vi "Stringfunction.vi"() -> ()   [LabVIEW 2020]
panel:
  out "decimated array 5":dbl[](array[numeric])
  out "decimated array 4":dbl[](array[numeric])
  out "decimated array 3":dbl[](array[numeric])
  out "decimated array 2":dbl[](array[numeric])
  out "decimated array":dbl[](array[numeric])
  out "interleaved array":dbl[](array[numeric])
  out "appended array":dbl[][](array[numeric])
  out "array w/ subset deleted":dbl[][](array[numeric])
  out "output array 4":dbl[][](array[numeric])
  out "output array":dbl[][](array[numeric])
  out "min index(es)":i32[](array[numeric])
  out "max index(es)":i32[](array[numeric])
  out "size(s)":i32[](array[numeric])
  out "output array 3":dbl[][](array[numeric])
  out "min value":dbl
  out "max value":dbl
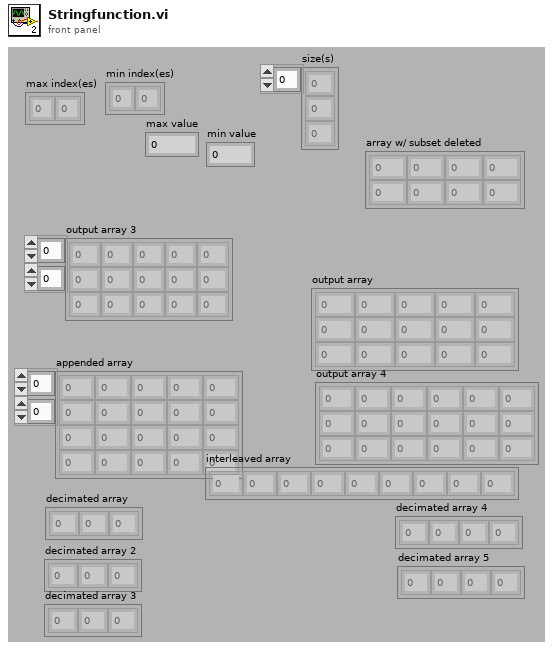
[diagram p1: front panel]
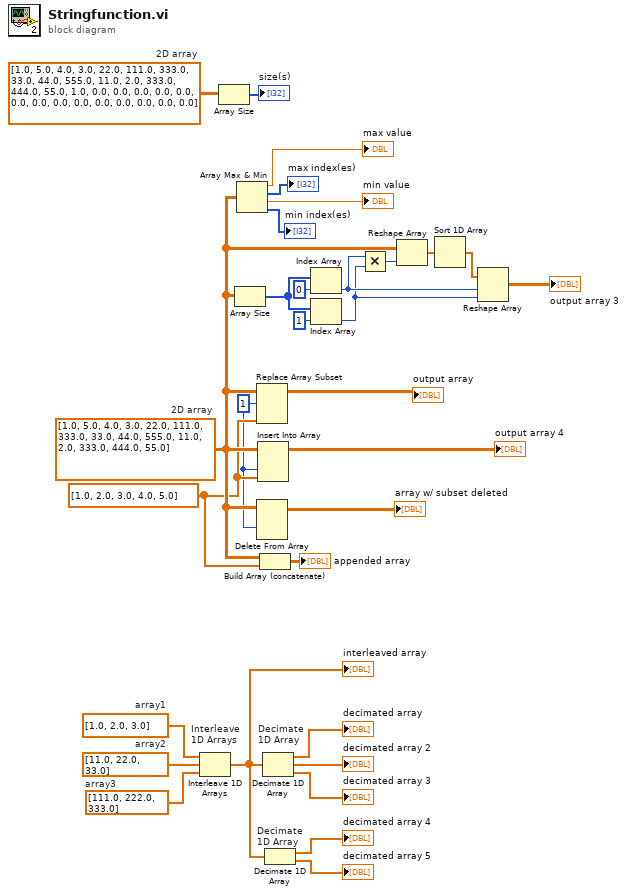
[diagram p0: block diagram]
diagram:
  w8 = dbl[] [111.0, 222.0, 333.0]  # array3
  w9 = dbl[] [11.0, 22.0, 33.0]  # array2
  w1 = dbl[] [1.0, 2.0, 3.0]  # array1
  w10 = 1 ("index (row)")
  w20 = dbl[][][] [[[1.0, 5.0, 4.0, 3.0, 22.0], [111.0, 333.0, 33.0, 44.0, 555.0], [11.0, 2.0, 333.0, 444.0, 55.0]], [[1.0, 0.0, 0.0, 0.0, 0.0], [0.0, 0.0, 0.0, 0.0, 0.0], [0.0, 0.0, 0.0, 0.0, 0.0]]]  # 2D array
  w12 = dbl[] [1.0, 2.0, 3.0, 4.0, 5.0] ("array")
  w13 = dbl[][] [[1.0, 5.0, 4.0, 3.0, 22.0], [111.0, 333.0, 33.0, 44.0, 555.0], [11.0, 2.0, 333.0, 444.0, 55.0]]  # 2D array
  n1 = Interleave 1D Arrays "Interleave\n1D Arrays"(w1, w9, w8) -> (w4:dbl[])
  "interleaved array" <- w4
  n2 = Array Size(array=w20) -> (size(s)=→"size(s)":i32[])
  n3 = Array Size(array=w13) -> (size(s)=w27:i32[])
  n4 = Array Max & Min(array=w13) -> (max value=→"max value":dbl, max index (indices)=→"max index(es)":i32[], min value=→"min value":dbl, min index (indices)=→"min index(es)":i32[])
  n5 = Replace Array Subset "Replace Array Subset"(array=w13, new element=w12, index (row)=w10) -> (→"output array":dbl[][])  [unwired: 1 in]
  n6 = Delete From Array "Delete From Array"(array=w13, index (row)=w10) -> (array with subset deleted=→"array w/ subset deleted":dbl[][])  [unwired: 2 in, 1 out]
  n7 = Insert Into Array "Insert Into Array"(array=w13, index (col)=w10, new element=w12) -> (→"output array 4":dbl[][])  [unwired: 1 in]
  n8 = Build Array (concatenate)(w13, w12) -> (→"appended array":dbl[][])
  n9 = Decimate 1D Array "Decimate\n1D Array"(w4) -> (→"decimated array":dbl[], →"decimated array 2":dbl[], →"decimated array 3":dbl[])
  n10 = Decimate 1D Array "Decimate\n1D Array"(w4) -> (→"decimated array 4":dbl[], →"decimated array 5":dbl[])
  n11 = Index Array "Index Array"(array=w27, index=0) -> (element=w23:i32)
  n12 = Index Array "Index Array"(array=w27, index=1) -> (element=w22:i32)
  n13 = Multiply(x=w23, y=w22) -> (x*y=w26:i32)
  n14 = Reshape Array "Reshape Array"(w13, w26) -> (w25:dbl[])
  n15 = Sort 1D Array(array=w25) -> (sorted array=w24:dbl[])
  n16 = Reshape Array "Reshape Array"(w24, w23, w22) -> (→"output array 3":dbl[][])
